vi "Get UI Path.vi"(10 "UI folder name":string) -> (2 "UI details":T1[](array[typedef]))   [LabVIEW 2021, in "Audio ADC Shared.lvlib"]
uses:
  Audio ADC Shared.lvlib
  <vilib>/MeasurementLink/MeasurementLink Measurement Server/Helpers/TypeDefs/User Interface Information.ctl
  <vilib>/MeasurementLink/MeasurementLink Measurement Server/MeasurementLink Measurement Server.lvlib
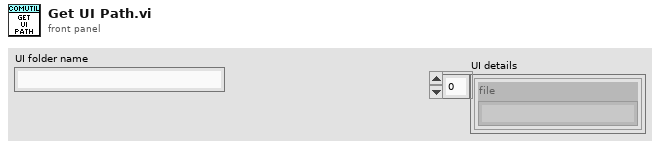
[diagram p1: front panel]
types:
  T1 = typedef "MeasurementLink Measurement Server.lvlib/User Interface Information.ctl" = cluster{"file":string}
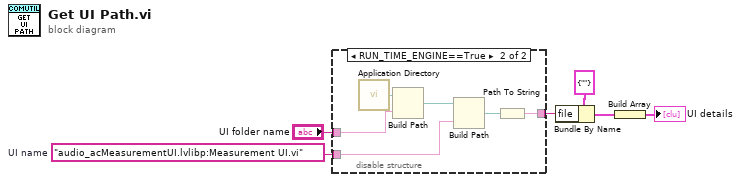
[diagram p0: block diagram]
diagram:
  w5 = "audio_acMeasurementUI.lvlibp:Measurement UI.vi"  # UI name
  n1 = disable-structure shown="RUN_TIME_ENGINE==True" {
    disable-tunnel: "UI folder name" -> [_ w13]
    disable-tunnel: w5 -> [w7 w11]
    disable-tunnel: [w7 w9] -> w2
    frame condition #0 (active) {
    }
    frame condition #1 {
      n2 = call <vilib>:"Application Directory.vi"() -> ("Application Directory"=w8:path)
      n3 = Build Path(base path=w8, name or relative path=w13) -> (appended path=w12:path)
      n4 = Build Path(base path=w12, name or relative path=w11) -> (appended path=w10:path)
      n5 = Path To String(path=w10) -> (string=w9:string)
    }
  }
  n6 = Bundle By Name(cluster=T1 {"file"=""} ("UI Information"), "file"=w2) -> (w3:T1)
  n7 = Build Array(w3) -> (→"UI details":T1[])
